vi "quaternion_to_transform.vi"(11 "Quaternion":dbl[](array[numeric])) -> (3 "Transform matrix":T1 format="%#_3f")   [LabVIEW 2013]
uses:
  <vilib>/Analysis/Matrix/Datatypes/RealMatrix.ctl
  norm_vec.vi
  <vilib>/Analysis/Matrix/NI_Matrix.lvlib
panel:
  # "Given a quaternion, return the  transform matrix (with no translation component.)"
  # "w"
  # "x1"
  # "x2"
  # "x3"
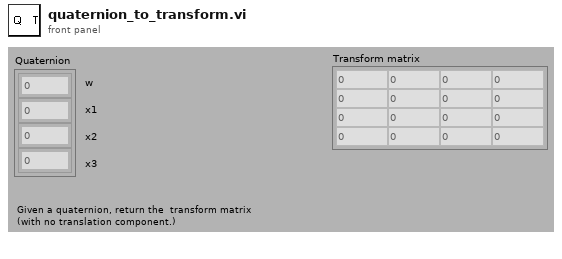
[diagram p1: front panel]
types:
  T1 = typedef "NI_Matrix.lvlib/RealMatrix.ctl" = dbl[][]
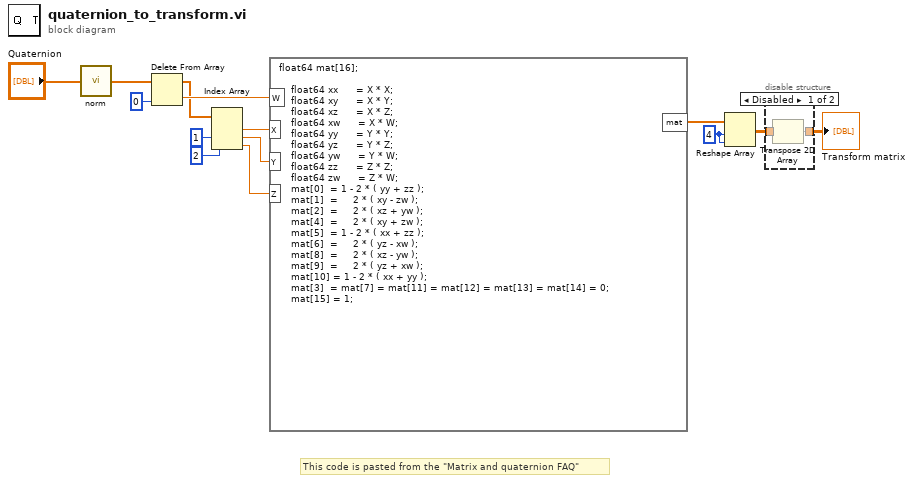
[diagram p0: block diagram]
diagram:
  w3 = 4 ("dimension size")
  # "This code is pasted from the \"Matrix and quaternion FAQ\""
  n1 = call-poly "norm.vi"("vector"="Quaternion") -> ("normalized vector"=w13:dbl[])  [unwired: 3 in, 1 out]
  n2 = Delete From Array(array=w13, index=0) -> (deleted portion=w11:dbl, array with subset deleted=w10:dbl[])  [unwired: 1 in]
  n3 = Index Array(array=w10, index #2=1 ("index"), index #3=2 ("index")) -> (element #1=w9:dbl, element #2=w8:dbl, element #3=w7:dbl)  [unwired: 1 in]
  n4 = formula code="float64 mat[16];\n\n    float64 xx      = X * X;\n    float64 xy      = X * Y;\n    float64 xz      = X * Z;\n    float64 xw      = X * W;\n    float64 yy      = Y * Y;\n    float64 yz      = Y * Z;\n    float64 yw      = Y * W;\n    float64 zz      = Z * Z;\n    float64 zw      = Z * W;\n    mat[0]  = 1 - 2 * ( yy + zz );\n    mat[1]  =     2 * ( xy - zw );\n    mat[2]  =     2 * ( xz + yw );\n    mat[4]  =     2 * ( xy + zw );\n    mat[5]  = 1 - 2 * ( xx + zz );\n    mat[6]  =     2 * ( yz - xw );\n    mat[8]  =     2 * ( xz - yw );\n    mat[9]  =     2 * ( yz + xw );\n    mat[10] = 1 - 2 * ( xx + yy );\n    mat[3]  = mat[7] = mat[11] = mat[12] = mat[13] = mat[14] = 0;\n    mat[15] = 1;"("W"=w11, "X"=w9, "Y"=w8, "Z"=w7) -> ("mat"=w4:dbl[])
  n5 = Reshape Array(w4, w3, w3) -> (w2:dbl[][])
  n6 = disable-structure shown="Disabled" {
    disable-tunnel: w2 -> [w16 w17]
    disable-tunnel: [w15 w17] -> w1
    frame Disabled {
      n7 = Transpose 2D Array(2D array=w16) -> (transposed array=w15:dbl[][])
    }
    frame Enabled {
    }
  }
  "Transform matrix" <- w1
